vi "Trigger.vi"   [LabVIEW 2013]
uses:
  <vilib>/Rock Robotics/WPI/Joystick/WPI_JoystickGetSetRefNum.vi
  Globals/Useful Values.vi
  Globals/Data for Dashboard.vi
types:
  T1 = typedef "WPI_JoystickDevRef.ctl" = cluster{"Device":T2}
  T2 = typedef "WPI_JoystickDeviceEnum.ctl" = enum16{"USB 1", "USB 2", "USB 3", "USB 4", "Kinect 1", "Kinect 2"}
  T3 = typedef "WPI_DigitalInputDevRef.ctl" = cluster{"DevStatus":errorcluster, "DIO Channel":T4, "Digital Module":T5}
  T4 = typedef "FPGA_DIOChannel.ctl" = enum8{"DIO 1", "DIO 2", "DIO 3", "DIO 4", "DIO 5", "DIO 6", "DIO 7", "DIO 8", "DIO 9", "DIO 10", "DIO 11", "DIO 12", "DIO 13", "DIO 14", "Invalid"}
  T5 = typedef "FPGA_TypedefDigitalModule.ctl" = enum16{"Digital Module 1", "Digital Module 2"}
  T6 = typedef "WPI_AnalogChannelDevRef.ctl" = cluster{"DevStatus":errorcluster, "Analog Module":T7, "Analog Channel":T8}
  T7 = typedef "FPGA_TypedefAnalogModule.ctl" = enum16{"Analog Module 1", "Analog Module 2"}
  T8 = typedef "FPGA_AIChannel.ctl" = enum8{"AI 1", "AI 2", "AI 3", "AI 4", "AI 5", "AI 6", "AI 7", "AI 8", "Invalid"}
  T9 = typedef "WPI_MotorControlDeviceRef.ctl" = cluster{"DeviceStatus":errorcluster, "Type":enum16{"PWM", "CAN"}, "PWM":cluster{"Digital Module":T5, "PWM Channel":T10, "DeadBand":T11}, "CAN":cluster{"Device Number":u8, "Control Mode":T12, "Semaphore":T13, "Max Vout":dbl}, "Invert":bool, "TransformRef":T14, "InvTransformRef":T14}
  T10 = typedef "FPGA_DIOPWMChannel.ctl" = enum8{"PWM 1", "PWM 2", "PWM 3", "PWM 4", "PWM 5", "PWM 6", "PWM 7", "PWM 8", "PWM 9", "PWM 10", "Invalid"}
  T11 = typedef "WPI_PWMDeadband.ctl" = cluster{"Name":string, "maxPositivePwm":i32, "minPositivePwm":i32, "centerPwm":i32, "maxNegativePwm":i32, "minNegativePwm":i32, "angularRange":u16}
  T12 = typedef "WPI_CANJaguar_ControlMode.ctl" = enum8{"Percent VBus", "Current", "Speed", "Position", "Voltage"}
  T13 = typedef "Semaphore RefNum" = refnum<k1>
  T14 = typedef "WPI_PWMTransform_ConPane.ctl" = refnum<vi>
  T15 = typedef "WPI_JoystickButtonState.ctl" = cluster{"Button 1":bool, "Button 2":bool, "Button 3":bool, "Button 4":bool, "Button 5":bool, "Button 6":bool, "Button 7":bool, "Button 8":bool, "Button 9":bool, "Button 10":bool, "Button 11":bool, "Button 12":bool}
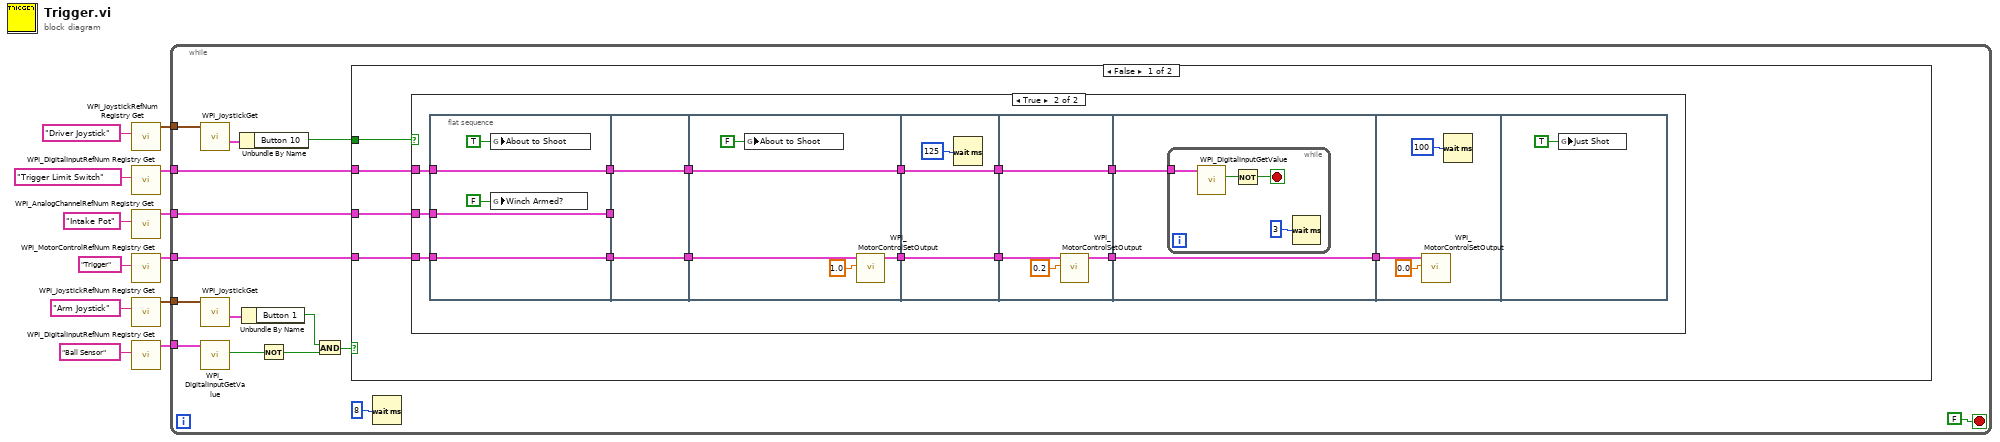
[diagram p0: block diagram]
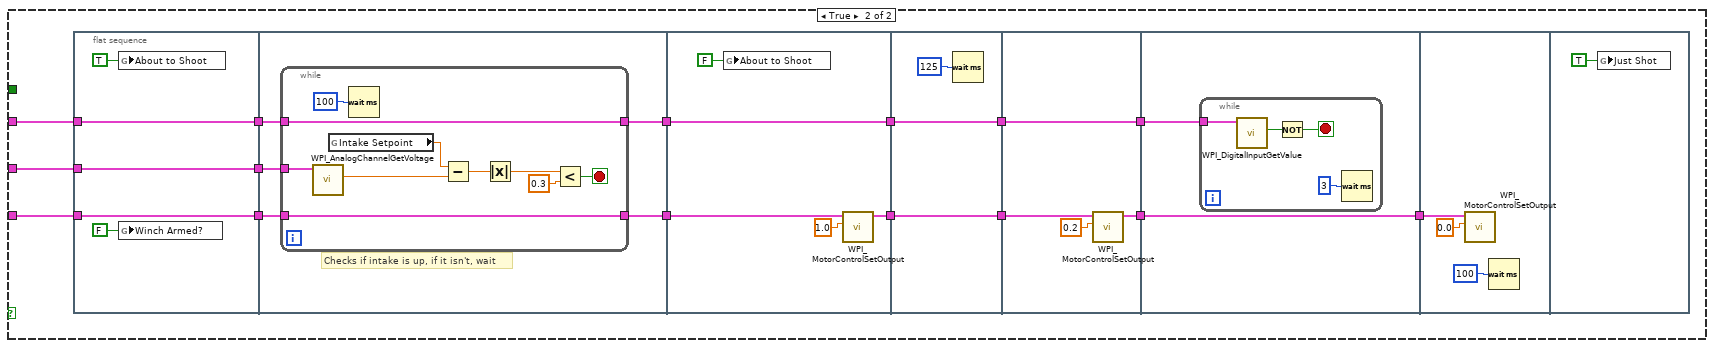
[diagram p3: hidden frame]
diagram:
  n1 = call <vilib>:"WPI_JoystickRefNum Registry Get.vi"("refnum name"="Driver Joystick") -> ("JoystickDevRef"=w3:T1)  [unwired: 9 in, 1 out]
  n2 = call <vilib>:"WPI_DigitalInputRefNum Registry Get.vi"("refnum name"="Trigger Limit Switch") -> ("DigitalInputDevRef"=w7:T3)  [unwired: 9 in, 1 out]
  n3 = call <vilib>:"WPI_AnalogChannelRefNum Registry Get.vi"("refnum name"="Intake Pot") -> ("AIDeviceRef"=w5:T6)  [unwired: 9 in, 1 out]
  n4 = call <vilib>:"WPI_MotorControlRefNum Registry Get.vi"("refnum name"="Trigger") -> ("MotorControlDevRef"=w9:T9)  [unwired: 9 in, 1 out]
  n5 = call <vilib>:"WPI_JoystickRefNum Registry Get.vi"("refnum name"="Arm Joystick") -> ("JoystickDevRef"=w11:T1)  [unwired: 9 in, 1 out]
  n6 = call <vilib>:"WPI_DigitalInputRefNum Registry Get.vi"("refnum name"="Ball Sensor") -> ("DigitalInputDevRef"=w1:T3)  [unwired: 9 in, 1 out]
  n7 = while {
    tunnel: w11 -> [w25]
    tunnel: w9 -> [w23]
    tunnel: w7 -> [w22]
    tunnel: w5 -> [w21]
    tunnel: w3 -> [w20]
    tunnel: w1 -> [w17]
    stop <- FALSE stop-if-true
    n8 = call <vilib>:"WPI_JoystickGet.vi"("JoystickDevRef"=w20) -> ("Buttons"=w19:T15)  [unwired: 4 in, 2 out]
    n9 = call <vilib>:"WPI_JoystickGet.vi"("JoystickDevRef"=w25) -> ("Buttons"=w24:T15)  [unwired: 4 in, 2 out]
    n10 = call <vilib>:"WPI_DigitalInputGetValue.vi"("DigitalInputDevRef"=w17) -> ("Value"=w14:bool)  [unwired: 8 in, 2 out]
    n11 = Unbundle By Name(w19) -> ("Button 10"=w18:bool)
    n12 = Unbundle By Name(w24) -> ("Button 1"=w15:bool)
    n13 = Not(x=w14) -> (.not. x?=w13:bool)
    n14 = And(x=w15, y=w13) -> (x .and. y?=w16:bool)
    n15 = case shown="False" w16 {
      tunnel: w22 -> [w29 w90]
      tunnel: w23 -> [w31 w84]
      tunnel: w21 -> [w28 w87]
      tunnel: w18 -> [w30 _]
      frame False {
        n16 = case shown="True" w30 {
          tunnel: w31 -> [_ w35]
          tunnel: w29 -> [_ w33]
          tunnel: w28 -> [_ w34]
          frame False {
          }
          frame True {
            n17 = flat-sequence {
              tunnel: w33 -> [w51]
              tunnel: [w51] -> w46
              tunnel: w34 -> [w49]
              tunnel: [w49] -> w45
              tunnel: w35 -> [w48]
              tunnel: [w48] -> w44
              tunnel: w46 -> [w53]
              tunnel: w45 -> [_]
              tunnel: [w53] -> w43
              tunnel: w44 -> [w52]
              tunnel: [w52] -> w32
              tunnel: w43 -> [w58]
              tunnel: [w58] -> w42
              tunnel: [w54] -> w41
              tunnel: w32 -> [w55]
              tunnel: w42 -> [w61]
              tunnel: [w61] -> w40
              tunnel: w41 -> [w60]
              tunnel: [w60] -> w39
              tunnel: [w65] -> w38
              tunnel: w40 -> [w65]
              tunnel: w39 -> [w63]
              tunnel: [w62] -> w37
              tunnel: w38 -> [w67]
              tunnel: w37 -> [w66]
              tunnel: [w66] -> w36
              tunnel: w36 -> [w72]
              frame #0 {
                n18 = global write "Useful Values.vi" "About to Shoot"(TRUE ("Just Shot")) -> ()
                n19 = global write "Data for Dashboard.vi" "Winch Armed?"(FALSE ("Winch Armed?")) -> ()
              }
              frame #1 {
              }
              frame #2 {
                n20 = global write "Useful Values.vi" "About to Shoot"(FALSE ("Just Shot")) -> ()
                n21 = call <vilib>:"WPI_MotorControlSetOutput.vi"("Output"=1.0 ("Motor Speed"), "MotorControlDevRef"=w55) -> ("MotorControlDevRef"=w54:T9)  [unwired: 7 in, 2 out]
              }
              frame #3 {
                n22 = Wait (ms)(milliseconds to wait=u32 125) -> ()  [unwired: 1 out]
              }
              frame #4 {
                n23 = call <vilib>:"WPI_MotorControlSetOutput.vi"("Output"=0.2 ("Motor Speed"), "MotorControlDevRef"=w63) -> ("MotorControlDevRef"=w62:T9)  [unwired: 7 in, 2 out]
              }
              frame #5 {
                n24 = while {
                  tunnel: w67 -> [w71]
                  stop <- w69 stop-if-true
                  n25 = call <vilib>:"WPI_DigitalInputGetValue.vi"("DigitalInputDevRef"=w71) -> ("Value"=w70:bool)  [unwired: 8 in, 2 out]
                  n26 = Not(x=w70) -> (.not. x?=w69:bool)
                  n27 = Wait (ms)(milliseconds to wait=u32 3) -> ()  [unwired: 1 out]
                }
              }
              frame #6 {
                n28 = call <vilib>:"WPI_MotorControlSetOutput.vi"("Output"=0.0 ("Motor Speed"), "MotorControlDevRef"=w72) -> ()  [unwired: 7 in, 3 out]
                n29 = Wait (ms)(milliseconds to wait=u32 100) -> ()  [unwired: 1 out]
              }
              frame #7 {
                n30 = global write "Useful Values.vi" "Just Shot"(TRUE ("Just Shot")) -> ()
              }
            }
          }
        }
      }
      frame True {
        n31 = flat-sequence {
          tunnel: w90 -> [w95]
          tunnel: [w95] -> w88
          tunnel: w87 -> [w93]
          tunnel: [w93] -> w86
          tunnel: w84 -> [w92]
          tunnel: [w92] -> w83
          tunnel: w88 -> [w99]
          tunnel: w86 -> [w100]
          tunnel: [w98] -> w85
          tunnel: w83 -> [w97]
          tunnel: [w96] -> w82
          tunnel: w85 -> [w115]
          tunnel: [w115] -> w81
          tunnel: w82 -> [w112]
          tunnel: [w111] -> w79
          tunnel: w81 -> [w118]
          tunnel: [w118] -> w80
          tunnel: w79 -> [w117]
          tunnel: [w117] -> w78
          tunnel: [w122] -> w89
          tunnel: w80 -> [w122]
          tunnel: w78 -> [w120]
          tunnel: [w119] -> w77
          tunnel: w89 -> [w124]
          tunnel: w77 -> [w123]
          tunnel: [w123] -> w76
          tunnel: w76 -> [w129]
          frame #0 {
            n32 = global write "Useful Values.vi" "About to Shoot"(TRUE ("Just Shot")) -> ()
            n33 = global write "Data for Dashboard.vi" "Winch Armed?"(FALSE ("Winch Armed?")) -> ()
          }
          frame #1 {
            # "Checks if intake is up, if it isn't, wait"
            n34 = while {
              tunnel: w100 -> [w110]
              tunnel: w99 -> [w107]
              tunnel: [w107] -> w98
              tunnel: w97 -> [w102]
              tunnel: [w102] -> w96
              stop <- w106 stop-if-true
              n35 = call <vilib>:"WPI_AnalogChannelGetVoltage.vi"("AIDeviceRef"=w110) -> ("Voltage"=w109:dbl)  [unwired: 8 in, 2 out]
              n36 = global read "Useful Values.vi" "Intake Setpoint"() -> (w103:dbl)
              n37 = Wait (ms)(milliseconds to wait=u32 100) -> ()  [unwired: 1 out]
              n38 = Subtract(x=w103, y=w109) -> (x-y=w108:dbl)
              n39 = Absolute Value(x=w108) -> (abs(x)=w104:dbl)
              n40 = Less?(x=w104, y=0.3) -> (x < y?=w106:bool)
            }
          }
          frame #2 {
            n41 = global write "Useful Values.vi" "About to Shoot"(FALSE ("Just Shot")) -> ()
            n42 = call <vilib>:"WPI_MotorControlSetOutput.vi"("Output"=1.0 ("Motor Speed"), "MotorControlDevRef"=w112) -> ("MotorControlDevRef"=w111:T9)  [unwired: 7 in, 2 out]
          }
          frame #3 {
            n43 = Wait (ms)(milliseconds to wait=u32 125) -> ()  [unwired: 1 out]
          }
          frame #4 {
            n44 = call <vilib>:"WPI_MotorControlSetOutput.vi"("Output"=0.2 ("Motor Speed"), "MotorControlDevRef"=w120) -> ("MotorControlDevRef"=w119:T9)  [unwired: 7 in, 2 out]
          }
          frame #5 {
            n45 = while {
              tunnel: w124 -> [w128]
              stop <- w126 stop-if-true
              n46 = call <vilib>:"WPI_DigitalInputGetValue.vi"("DigitalInputDevRef"=w128) -> ("Value"=w127:bool)  [unwired: 8 in, 2 out]
              n47 = Not(x=w127) -> (.not. x?=w126:bool)
              n48 = Wait (ms)(milliseconds to wait=u32 3) -> ()  [unwired: 1 out]
            }
          }
          frame #6 {
            n49 = call <vilib>:"WPI_MotorControlSetOutput.vi"("Output"=0.0 ("Motor Speed"), "MotorControlDevRef"=w129) -> ()  [unwired: 7 in, 3 out]
            n50 = Wait (ms)(milliseconds to wait=u32 100) -> ()  [unwired: 1 out]
          }
          frame #7 {
            n51 = global write "Useful Values.vi" "Just Shot"(TRUE ("Just Shot")) -> ()
          }
        }
      }
    }
    n52 = Wait (ms)(milliseconds to wait=u32 8) -> ()  [unwired: 1 out]
  }
